vi "GetType.vi"(8 "error in (no error)":errorcluster, 11 "ReferenceMove Msg":refnum<class "ReferenceMove Msg.lvclass">) -> (0 "error out":errorcluster, 2 "Data Sample":variant, 3 "ReferenceMove Msg":refnum<class "ReferenceMove Msg.lvclass">)   [LabVIEW 2015, in "CS++Motor.lvlib" / "ReferenceMove Msg.lvclass"]
uses:
  ReferenceMove Msg.lvclass
  ReferenceMove Msg.lvclass/ReferenceMove Msg.ctl
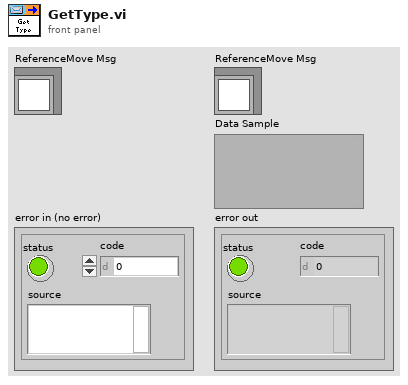
[diagram p1: front panel]
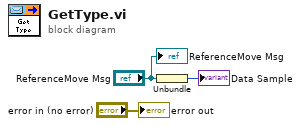
[diagram p0: block diagram]
diagram:
  n1 = Unbundle("ReferenceMove Msg") -> (→"Data Sample":u8)
  "error out" <- "error in (no error)"
  "ReferenceMove Msg" <- "ReferenceMove Msg"
